vi "Gabor Filter (Mask).vi"(8 "error in (no error)":errorcluster, 9 "mask array":bool[][](array[boolean]), 10 "dest RefNum in":T1, 11 "src RefNum in":T1) -> (0 "error out":errorcluster, 2 "dest RefNum out":T1, 3 "RefNum out":T1)   [LabVIEW 2017, in "SoundVib_Gabor.lvlib"]
doc: "Removes the Gabor coefficients from the data block referenced by <B>src RefNum in</B> that are outside the mask and stores the result in a data block referenced by <B>dest RefNum out</B>."
uses:
  <vilib>/addons/Sound and Vibration/Order Analysis/Gabor Order Tracking/SoundVib_Gabor.lvlib
  <vilib>/addons/Sound and Vibration/Order Analysis/Ref Gabor Order Tracking/GT RefNum.ctl
  <resource>/sndvib.dll
panel:
  # "Gabor Filter (Mask)"
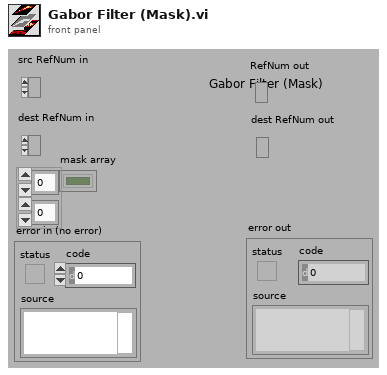
[diagram p1: front panel]
types:
  T1 = typedef "SoundVib_Gabor.lvlib/GT RefNum.ctl" = refnum<k1>
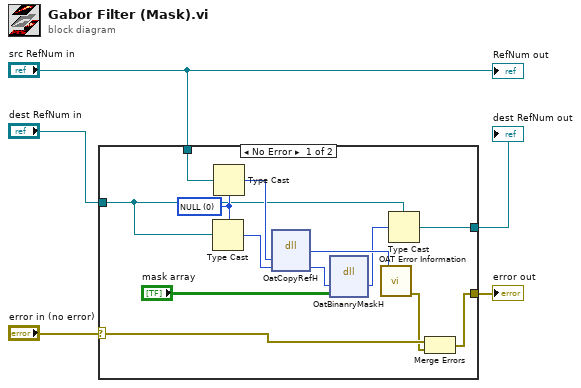
[diagram p0: block diagram]
diagram:
  n1 = case shown="No Error" "error in (no error)" {
    selector: "error in (no error)" -> [w8 w20]
    tunnel: [w6 w20] -> w5
    tunnel: "src RefNum in" -> [w14 _]
    tunnel: "dest RefNum in" -> [w10 w19]
    tunnel: [w9 w19] -> w1
    frame No Error {
      w17 = u32 0 items=["NULL"]
      n2 = Type Cast(type=w17, x=w10) -> (*(type *) &x=w16:u32)
      n3 = Type Cast(type=w17, x=w14) -> (*(type *) &x=w18:u32)
      n4 = dll-call lib="C:/Program Files (x86)/National Instruments/LabVIEW 2017/resource/sndvib.*" fn="OatCopyRefH"("Ref Src"=w18, "Ref Masked"=w16) -> ("return type"=w15:i32, "Ref Masked"=w13:u32)  [unwired: 4 in, 2 out]
      n5 = dll-call lib="C:/Program Files (x86)/National Instruments/LabVIEW 2017/resource/sndvib.*" fn="OatBinanryMaskH"("RefSrc"=w13, "Mask"="mask array") -> ("RefSrc"=w11:u32)  [unwired: 5 in, 2 out]
      n6 = call <vilib>:"OAT Error Information.vi"("error code"=w15) -> ("error out"=w7:errorcluster)  [unwired: 6 in]
      n7 = Type Cast(type=w10, x=w11) -> (*(type *) &x=w9:T1)
      n8 = Merge Errors(w8, w7) -> (w6:errorcluster)
    }
    frame Error {
    }
  }
  "error out" <- w5
  "dest RefNum out" <- w1
  "RefNum out" <- "src RefNum in"
